vi "wind-rotor-ratio-3.vi"() -> ()   [LabVIEW 2009]
uses:
  <vilib>/express/express arith-compare/Formula/XNode/ExpressFormulaBlockNode.xnode
panel:
  out "Buffered Data":dbl[][](array[numeric])
  in  "end program":bool
  in  "Wind direction (deg)":dbl(knob) step=1.0 scale=0.0..360.0
  in  "rotor speed (rpm)":dbl(knob) scale=0.0..250.0
  in  "Wind speed (m/s)":dbl(knob) scale=0.0..30.0
  out "wind/rotor-ratio":picture
  in  "Settings":T1={"maximum"=0.0, "minimum"=0.0, "clip to min"=FALSE, "log?(F)"=FALSE, "grid color"=6710886, "plot color"=65280, "fmt and prec"={"format"=enum."Decimal", "precision"=0}, "visible section"=8} {"minimum" format="%0.2f"; "maximum" format="%0.2f"}
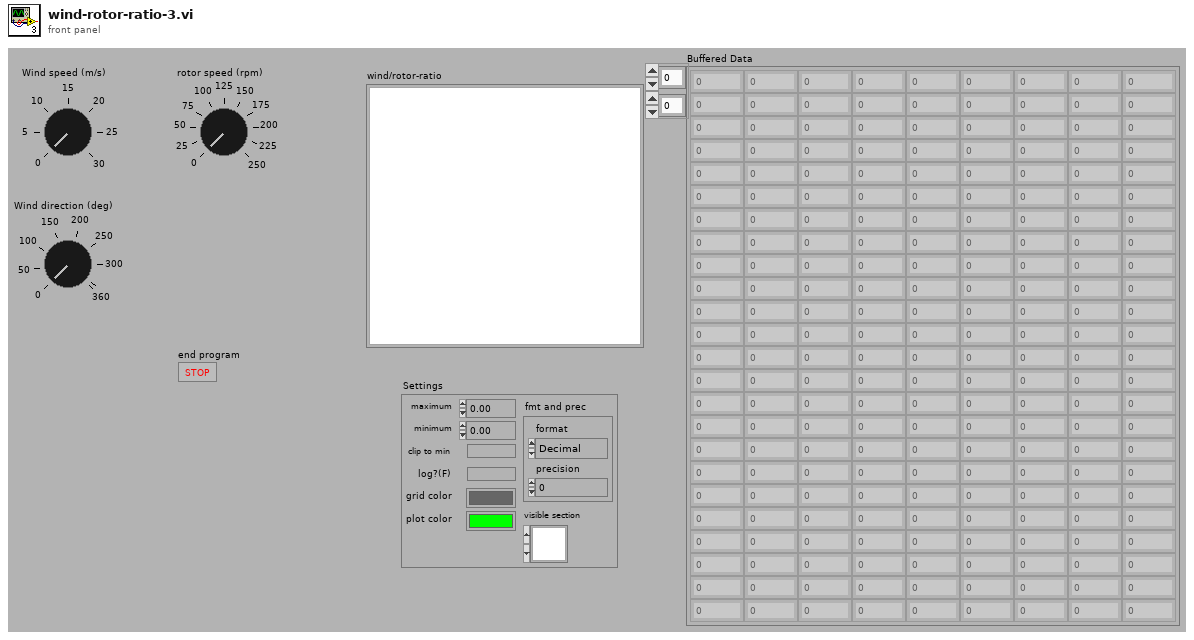
[diagram p1: front panel]
types:
  T1 = cluster{"maximum":dbl, "minimum":dbl, "clip to min":bool, "log?(F)":bool, "grid color":u32, "plot color":u32, "fmt and prec":cluster{"format":enum8{"Decimal", "Scientific", "Engineering", "Binary", "Octal", "Hex"}, "precision":u8}, "visible section":u16}
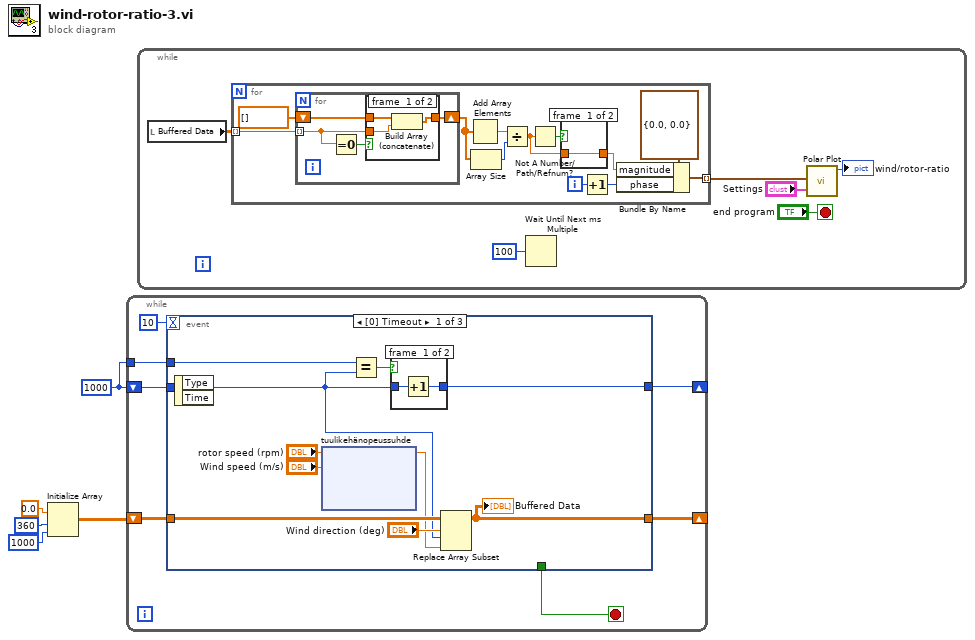
[diagram p0: block diagram]
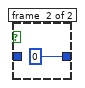
[diagram p2: hidden frame]
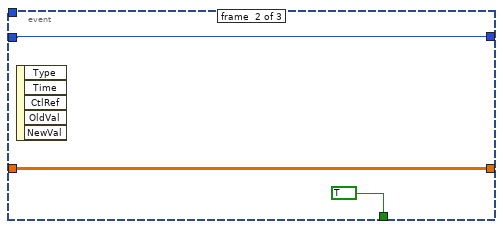
[diagram p3: hidden frame]
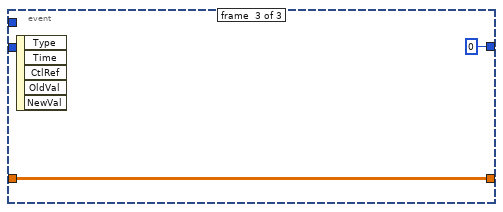
[diagram p4: hidden frame]
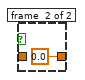
[diagram p5: hidden frame]
diagram:
  w2 = 1000
  n1 = Initialize Array(0.0, 360 ("dimension size"), 1000 ("dimension size")) -> (w1:dbl[][])
  n2 = while {
    shift-right: [w10] -> _
    shift-left: w1 -> [w12]
    shift-right: [w11] -> _
    shift-left: w2 -> [w9]
    tunnel: w2 -> [w8]
    stop <- w7 stop-if-true
    n3 = event shown="[0] Timeout" {
      selector: _ -> [_ _ _]
      dyn-events: _ -> [_ _ _]
      timeout: 10 -> [_ _ _]
      tunnel: w12 -> [w21 w37 w39]
      tunnel: [w19 w36 0] -> w11
      tunnel: [w18 w37 w39] -> w10
      tunnel: w9 -> [w17 w36 _]
      tunnel: w8 -> [w16 _ _]
      tunnel: [_ TRUE _] -> w7
      event #0 {
        n4 = event-data() -> ()  [unwired: 1 in, 2 out]
        n5 = xnode "tuulikehänopeussuhde"("X1"="rotor speed (rpm)", "X2"="Wind speed (m/s)") -> ("Result"=w20:dbl)  [unwired: 1 in, 1 out]
        n6 = Equal?(x=w16, y=w17) -> (x = y?=w15:bool)
        n7 = case shown="False" w15 {
          tunnel: w17 -> [w24 _]
          tunnel: [w23 0] -> w19
          frame #0 {
            n8 = Increment(x=w24) -> (x+1=w23:i32)
          }
          frame #1 {
          }
        }
        n9 = Replace Array Subset(array=w21, new element=w20, index (row)="Wind direction (deg)", index (col)=w17) -> (w18:dbl[][])
        "Buffered Data" <- w18
      }
      event #1 {
        n10 = event-data() -> ()  [unwired: 1 in, 5 out]
      }
      event #2 {
        n11 = event-data() -> ()  [unwired: 1 in, 5 out]
      }
    }
  }
  n12 = while {
    stop <- "end program" stop-if-true
    n13 = local read "Buffered Data"() -> (w42:dbl[][])
    n14 = for {
      tunnel: w42 -> [w53] mode=indexing
      tunnel: [w54] -> w41 mode=indexing
      i -> [w56]
      n15 = for {
        tunnel: w53 -> [w62] mode=indexing
        shift-right: [w63] -> w51
        shift-left: dbl[] [] -> [w64]
        n16 = Equal To 0?(x=w62) -> (x = 0?=w61:bool)
        n17 = case shown="False" w61 {
          tunnel: w64 -> [w67 w68]
          tunnel: w62 -> [w66 _]
          tunnel: [w65 w68] -> w63
          frame #0 {
            n18 = Build Array (concatenate)(w67, w66) -> (w65:dbl[])
          }
          frame #1 {
          }
        }
      }
      n19 = Add Array Elements(numeric array=w51) -> (sum=w58:dbl)
      n20 = Array Size(array=w51) -> (size(s)=w57:i32)
      n21 = Divide(x=w58, y=w57) -> (x/y=w49:dbl)
      n22 = Not A Number/Path/Refnum?(number/path/refnum=w49) -> (NaN/Path/Refnum?=w50:bool)
      n23 = case shown="True" w50 {
        tunnel: w49 -> [w59 _]
        tunnel: [w59 0.0] -> w47
        frame #0 {
        }
        frame #1 {
        }
      }
      n24 = Increment(x=w56) -> (x+1=w48:i32)
      n25 = Bundle By Name(cluster=cluster{"magnitude":dbl, "phase":dbl} {"magnitude"=0.0, "phase"=0.0}, "magnitude"=w47, "phase"=w48) -> (w54:cluster{"magnitude":dbl, "phase":dbl})
    }
    n26 = Wait Until Next ms Multiple(millisecond multiple=u32 100) -> ()  [unwired: 1 out]
    n27 = call <vilib>:"Polar Plot.vi"("polar attributes"="Settings", "data array [mag, phase (deg)]"=w41) -> ("new picture"=→"wind/rotor-ratio":picture)  [unwired: 9 in]
  }
